vi "Finish.vi"   [LabVIEW 2020]
doc: "This VI is called during exit. It can be used to close I/O refnums, save collected data, etc."
uses:
  <vilib>/Rock Robotics/WPI/Utilities/WPI_GetSetVariantRefNum.vi
types:
  T1 = typedef "WPI_CompressorDevRef.ctl" = cluster{"DevStatus":errorcluster, "Pneumatics Control Module":u8}
  T2 = typedef "WPI_JoystickDevRef.ctl" = cluster{"Device":T3}
  T3 = typedef "WPI_JoystickDeviceEnum.ctl" = enum16{"USB 0", "USB 1", "USB 2", "USB 3", "USB 4", "USB 5"}
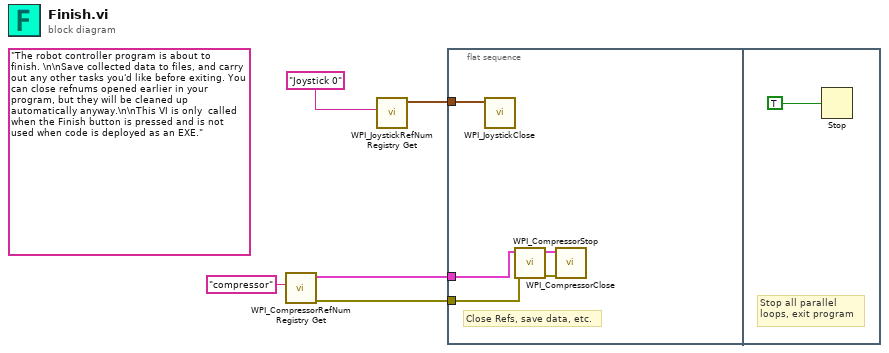
[diagram p0: block diagram]
diagram:
  (unwired) "The robot controller program is about to finish. \n\nSave collected data to files, and carry out any other tasks you'd like before exiting. You can close refnums opened earlier in your program, but they will be cleaned up automatically anyway.\n\nThis VI is only  called when the Finish button is pressed and is not used when code is deployed as an EXE."
  n1 = call <vilib>:"WPI_CompressorRefNum Registry Get.vi"("refnum name"="compressor") -> ("error out"=w1:errorcluster, "CompressorDevRef"=w2:T1)  [unwired: 9 in]
  n2 = call <vilib>:"WPI_JoystickRefNum Registry Get.vi"("refnum name"="Joystick 0") -> ("JoystickDevRef"=w4:T2)  [unwired: 1 in, 9 out]
  n3 = flat-sequence {
    tunnel: w4 -> [w10]
    tunnel: w2 -> [w9]
    tunnel: w1 -> [w8]
    frame #0 {
      # "Close Refs, save data, etc."
      n4 = call <vilib>:"WPI_JoystickClose.vi"("JoystickDevRef"=w10) -> ()  [unwired: 11 out]
      n5 = call <vilib>:"WPI_CompressorStop.vi"("error in (no error)"=w8, "CompressorDevRef"=w9) -> ("error out"=w7:errorcluster, "CompressorDevRef"=w6:T1)  [unwired: 8 in]
      n6 = call <vilib>:"WPI_CompressorClose.vi"("error in (no error)"=w7, "CompressorDevRef"=w6) -> ()  [unwired: 9 in, 1 out]
    }
    frame #1 {
      # "Stop all parallel\nloops, exit program"
      n7 = Stop(stop? (T)=TRUE ("Quit")) -> ()
    }
  }
